vi "Write LNA Gain dB.vi"(8 "error in (no error)":errorcluster, 10 "LNA Gain dB":dbl(knob)=4.5152468054049395 scale=0.0..50.0, 11 "HRF_Device in":refnum<class "HRF_Device.lvclass">) -> (0 "error out":errorcluster, 3 "HRF_Device out":refnum<class "HRF_Device.lvclass">)   [LabVIEW 2020, in "HRF_Device.lvclass"]
uses:
  HRF_Device.lvclass
  HRF_Device.lvclass/HRF_Device.ctl
  D:/work/HackRF/Labview Driver/NetHackrf.dll
  NetHackrf.dll
  Read Device ref.vi
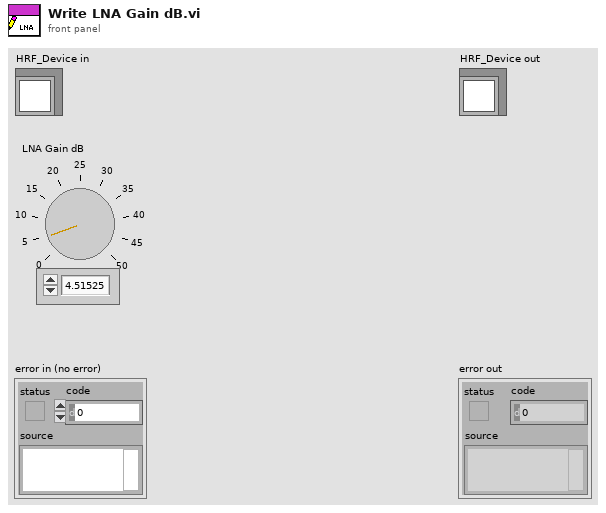
[diagram p1: front panel]
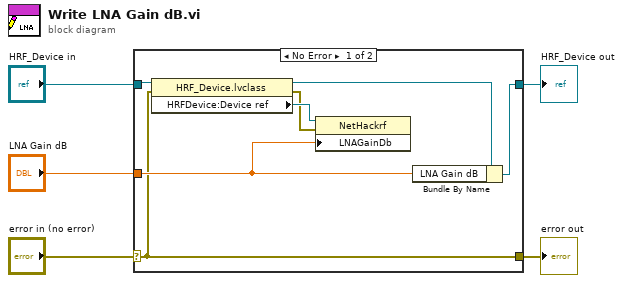
[diagram p0: block diagram]
diagram:
  n1 = case shown="No Error" "error in (no error)" {
    selector: "error in (no error)" -> [w7 w13]
    tunnel: [w7 w13] -> w4
    tunnel: [w12 w14] -> w2
    tunnel: "HRF_Device in" -> [w11 w14]
    tunnel: "LNA Gain dB" -> [w8 _]
    frame No Error {
      n2 = property class="HRF_Device.lvclass"(reference=w11, error in=w7) -> (reference out=w10:refnum<class "HRF_Device.lvclass">, error out=w6:errorcluster, "HRFDevice:Device ref"=w9:refnum<k24>)
      n3 = property class="NetHackrf"(reference=w9, error in=w6, "LNAGainDb"=w8) -> ()  [unwired: 2 out]
      n4 = Bundle By Name(cluster=w10, "LNA Gain dB"=w8) -> (w12:refnum<class "HRF_Device.lvclass">)
    }
    frame Error {
    }
  }
  "error out" <- w4
  "HRF_Device out" <- w2
